vi "Insect_circle_draw.vi"(1 "XYGraph in 2":refnum<vi>, 2 "XYGraph in":refnum<vi>, 3 "appended array":dbl[][](array[numeric])) -> (0 "Array":cluster{dbl[], dbl[]}[](array[cluster]))   [LabVIEW 2023]
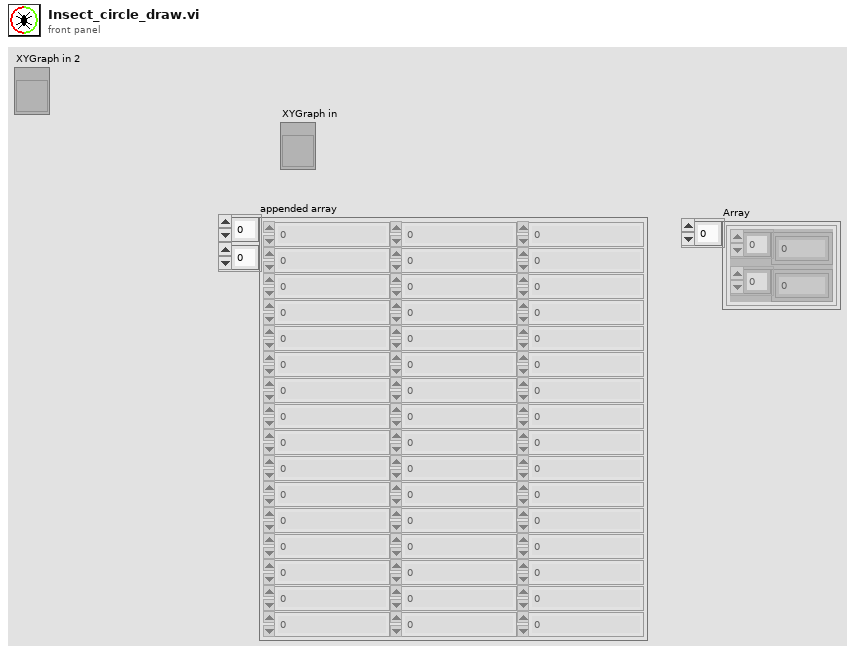
[diagram p1: front panel]
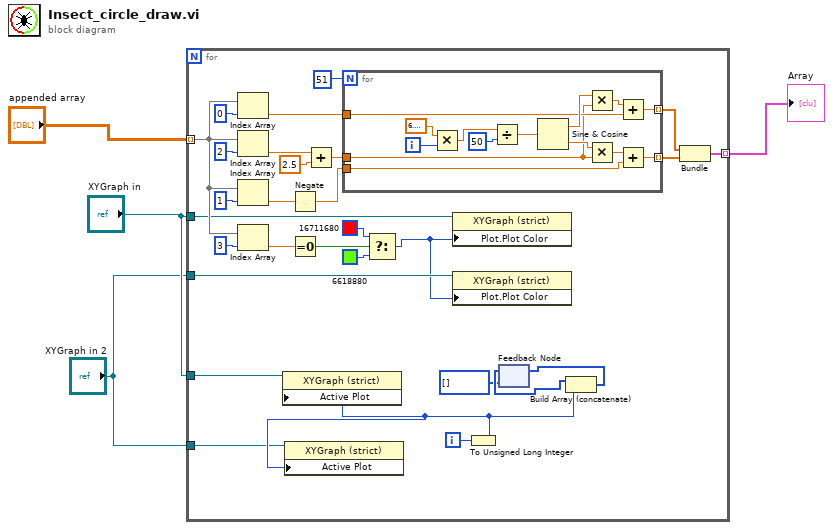
[diagram p0: block diagram]
diagram:
  n1 = for {
    tunnel: [w30] -> w3 mode=indexing
    tunnel: "appended array" -> [w21] mode=indexing
    tunnel: "XYGraph in" -> [w14]
    tunnel: "XYGraph in" -> [w13]
    tunnel: "XYGraph in 2" -> [w8]
    tunnel: "XYGraph in 2" -> [w5]
    i -> [w12]
    n2 = Index Array(array=w21, index=0) -> (element=w20:dbl)
    n3 = Index Array(array=w21, index=2) -> (element=w16:dbl)
    n4 = Index Array(array=w21, index=1) -> (element=w19:dbl)
    n5 = Index Array(array=w21, index=3) -> (element=w26:dbl)
    n6 = Negate(x=w19) -> (-x=w18:dbl)
    n7 = Equal To 0?(x=w26) -> (x = 0?=w25:bool)
    n8 = Add(x=w16, y=2.5) -> (x+y=w15:dbl)
    n9 = for {
      N: 51 ("Number of Points") -> [_]
      tunnel: [w41] -> w32 mode=indexing
      tunnel: [w40] -> w33 mode=indexing
      tunnel: w20 -> [w39]
      tunnel: w18 -> [w38]
      tunnel: w15 -> [w37]
      i -> [w47]
      n10 = Multiply(x=6.283185307179586, y=w47) -> (x*y=w36:dbl)
      n11 = Divide(x=w36, y=50) -> (x/y=w35:dbl)
      n12 = Sine & Cosine(0:w35) -> (1:w45:dbl, 2:w44:dbl)
      n13 = Multiply(x=w45, y=w37) -> (x*y=w43:dbl)
      n14 = Multiply(x=w44, y=w37) -> (x*y=w42:dbl)
      n15 = Add(x=w43, y=w39) -> (x+y=w41:dbl)
      n16 = Add(x=w42, y=w38) -> (x+y=w40:dbl)
    }
    n17 = Select(t=u32 16711680 ("Plot.Plot Color"), s=w25, f=u32 6618880 ("Plot.Plot Color")) -> (s? t:f=w7:u32)
    n18 = property on="Property Node" class="XYGraph (strict)"(reference=w13, "Plot.Plot Color"=w7) -> ()  [unwired: 1 in, 2 out]
    n19 = property on="Property Node" class="XYGraph (strict)"(reference=w8, "Plot.Plot Color"=w7) -> ()  [unwired: 1 in, 2 out]
    n20 = To Unsigned Long Integer(number=w12) -> (unsigned 32bit integer=w6:u32)
    n21 = property on="Property Node" class="XYGraph (strict)"(reference=w14, "Active Plot"=w6) -> ()  [unwired: 1 in, 2 out]
    n22 = property on="Property Node" class="XYGraph (strict)"(reference=w5, "Active Plot"=w6) -> ()  [unwired: 1 in, 2 out]
    n23 = feedback #1(u32[] []) -> (w10:u32[])
    n24 = Build Array (concatenate)(w10, w6) -> (w11:u32[])
    n25 = feedback-in #1(w11) -> ()
    n26 = Bundle(w32, w33) -> (w30:cluster{dbl[], dbl[]})  [unwired: 1 in]
  }
  "Array" <- w3
